vi "DB List Columns.vi"(8 "error in (no error)":errorcluster, 10 "table":string, 11 "MYSQL Database in":refnum<class "MYSQL Server.lvclass">) -> (0 "error out":errorcluster, 1 "tableDetails":string[][](array[string]), 2 "columns":string[](array[string]), 3 "MYSQL Database out":refnum<class "MYSQL Server.lvclass">)   [LabVIEW 2023, in "HardwareAbstractionLayer_LVOOP.lvlib" / "MYSQL Server.lvclass"]
uses:
  MYSQL Server.lvclass
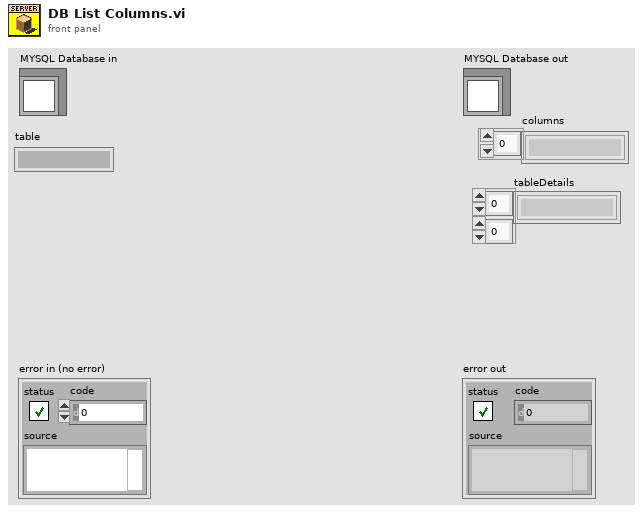
[diagram p1: front panel]
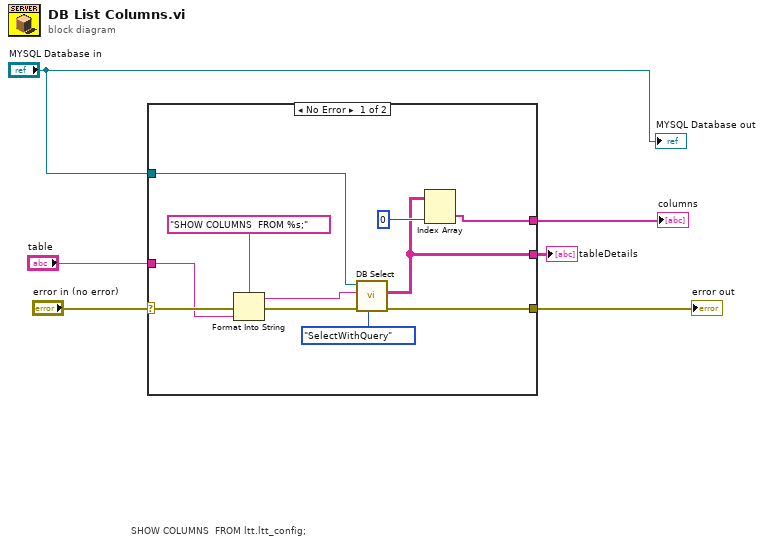
[diagram p0: block diagram]
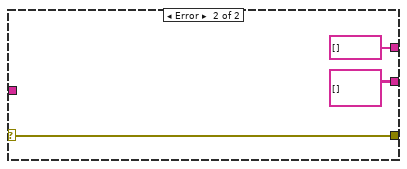
[diagram p2: hidden frame]
diagram:
  # "SHOW COLUMNS  FROM ltt.ltt_config;"
  n1 = case shown="No Error" "error in (no error)" {
    selector: "error in (no error)" -> [w14 w20]
    tunnel: "MYSQL Database in" -> [w17 _]
    tunnel: "table" -> [w12 _]
    tunnel: [w10 string[] [] ("columns")] -> w3
    tunnel: [w16 w20] -> w2
    tunnel: [w8 string[][] [] ("data")] -> w1
    frame No Error {
      n2 = Format Into String(format string="SHOW COLUMNS  FROM %s;", error in=w14, w12) -> (resulting string=w11:string, error out=w13:errorcluster)  [unwired: 1 in]
      n3 = call-dynamic "DB Select.vi"("Select"=enum16{"SelectWithQuery", "SelectWithColumn"}."SelectWithQuery", "error in (no error)"=w13, "SQL query"=w11, "Database in"=w17) -> ("error out"=w16:errorcluster, "data"=w8:string[][])  [unwired: 5 in, 1 out]
      n4 = Index Array(array=w8, index (col)=0 ("disabled index (col)")) -> (element=w10:string[])  [unwired: 1 in]
    }
    frame Error {
    }
  }
  "error out" <- w2
  "columns" <- w3
  "tableDetails" <- w1
  "MYSQL Database out" <- "MYSQL Database in"
